vi "Read Spec Page Path.vi"(8 "error in (no error)":errorcluster, 11 "PluginGenerator_MetaDataObj in":refnum<class "PluginGenerator_MetaDataObj.lvclass">) -> (0 "error out":errorcluster, 2 "Path to Spec Page VI":path, 3 "PluginGenerator_MetaDataObj out":refnum<class "PluginGenerator_MetaDataObj.lvclass">)   [LabVIEW 2023, in "Plugin Generator.lvlib" / "PluginGenerator_MetaDataObj.lvclass"]
uses:
  PluginGenerator_MetaDataObj.lvclass
  SpecPage.vi
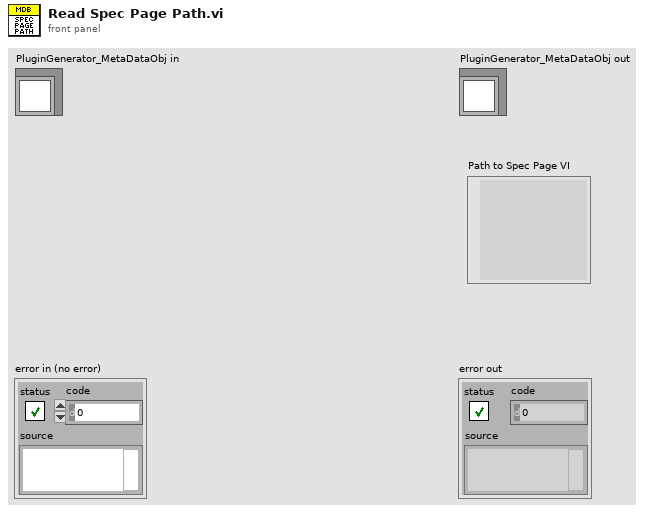
[diagram p1: front panel]
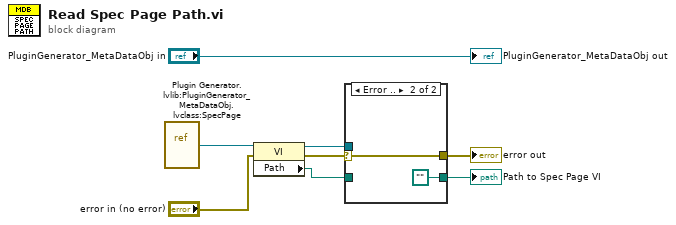
[diagram p0: block diagram]
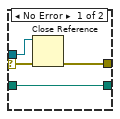
[diagram p2: hidden frame]
diagram:
  n1 = vi-ref "Plugin Generator.lvlib:PluginGenerator_MetaDataObj.lvclass:SpecPage.vi"() -> (w7:refnum<vi>)
  n2 = property class="VI"(reference=w7, error in="error in (no error)") -> (reference out=w6:refnum<vi>, error out=w4:errorcluster, "Path"=w1:path)
  n3 = case shown="Error .." w4 {
    selector: w4 -> [w11 w14]
    tunnel: w6 -> [w12 _]
    tunnel: [w10 w14] -> w3
    tunnel: [w9 path ""] -> w2
    tunnel: w1 -> [w9 _]
    frame No Error {
      n4 = Close Reference(reference=w12, error in (no error)=w11) -> (error out=w10:errorcluster)
    }
    frame Error {
    }
  }
  "error out" <- w3
  "Path to Spec Page VI" <- w2
  "PluginGenerator_MetaDataObj out" <- "PluginGenerator_MetaDataObj in"
